vi "PSK 2 bit par symbole.vi"() -> ()   [LabVIEW 2010]
panel:
  out "signal demodulé":bool[](array[boolean])
  out "Signal Modulé":dynamicdata(graph)
  in  "Tableau":bool[](array[boolean])
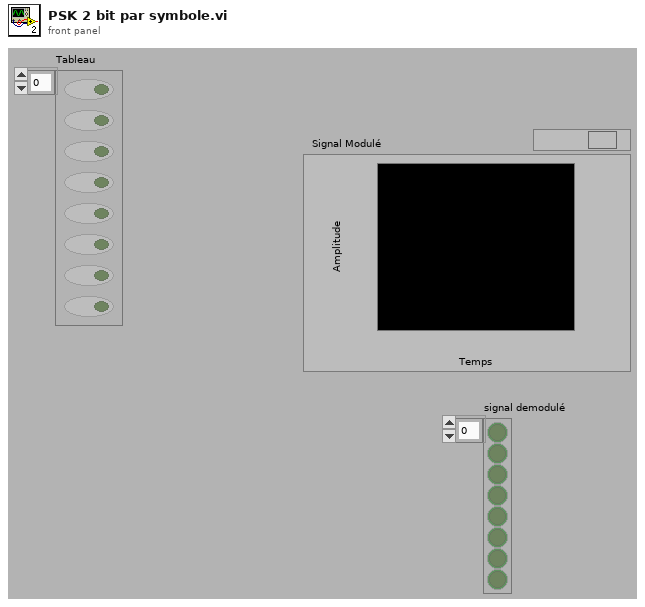
[diagram p1: front panel]
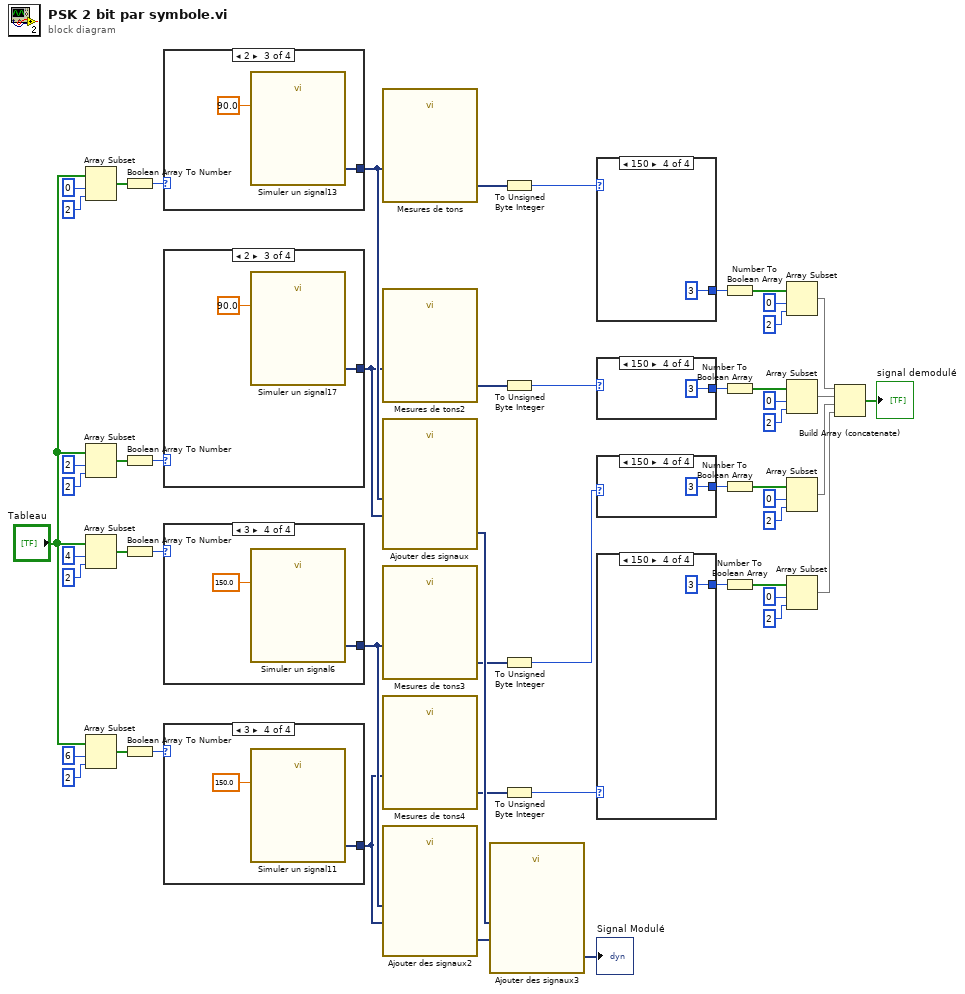
[diagram p0: block diagram]
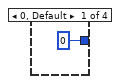
[diagram p2: hidden frame]
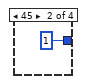
[diagram p3: hidden frame]
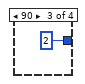
[diagram p4: hidden frame]
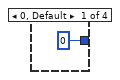
[diagram p5: hidden frame]
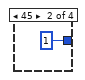
[diagram p6: hidden frame]
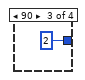
[diagram p7: hidden frame]
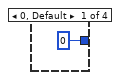
[diagram p8: hidden frame]
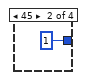
[diagram p9: hidden frame]
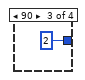
[diagram p10: hidden frame]
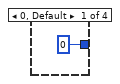
[diagram p11: hidden frame]
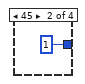
[diagram p12: hidden frame]
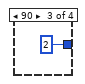
[diagram p13: hidden frame]
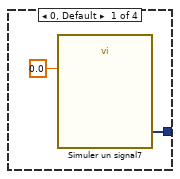
[diagram p14: hidden frame]
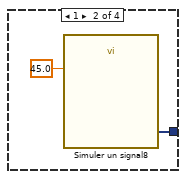
[diagram p15: hidden frame]
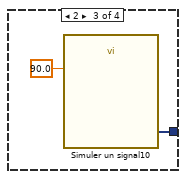
[diagram p16: hidden frame]
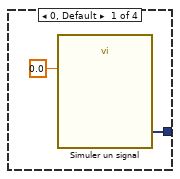
[diagram p17: hidden frame]
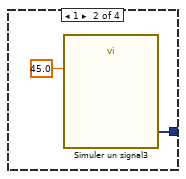
[diagram p18: hidden frame]
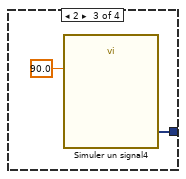
[diagram p19: hidden frame]
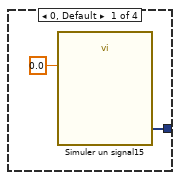
[diagram p20: hidden frame]
diagram:
  n1 = Array Subset(array="Tableau", index=0 ("indice"), length=2 ("longueur")) -> (w44:bool[])
  n2 = Array Subset(array="Tableau", index=2 ("indice"), length=2 ("longueur")) -> (w43:bool[])
  n3 = Array Subset(array="Tableau", index=4 ("indice"), length=2 ("longueur")) -> (w42:bool[])
  n4 = Array Subset(array="Tableau", index=6 ("indice"), length=2 ("longueur")) -> (w41:bool[])
  n5 = Boolean Array To Number(Boolean array=w44) -> (number=w40:u32)
  n6 = Boolean Array To Number(Boolean array=w43) -> (number=w38:u32)
  n7 = Boolean Array To Number(Boolean array=w42) -> (number=w36:u32)
  n8 = Boolean Array To Number(Boolean array=w41) -> (number=w35:u32)
  n9 = case shown="2" w40 {
    tunnel: [w54 w56 w58 w60] -> w33
    frame 0, Default {
      n10 = call "Simuler un signal5"("Phase"=0.0) -> ("Sinus"=w54:dynamicdata)  [unwired: 13 in, 1 out]
    }
    frame 1 {
      n11 = call "Simuler un signal9"("Phase"=45.0) -> ("Sinus"=w56:dynamicdata)  [unwired: 13 in, 1 out]
    }
    frame 2 {
      n12 = call "Simuler un signal13"("Phase"=90.0) -> ("Sinus"=w58:dynamicdata)  [unwired: 13 in, 1 out]
    }
    frame 3 {
      n13 = call "Simuler un signal2"("Phase"=150.0) -> ("Sinus"=w60:dynamicdata)  [unwired: 13 in, 1 out]
    }
  }
  n14 = case shown="2" w38 {
    tunnel: [w62 w64 w66 w68] -> w31
    frame 0, Default {
      n15 = call "Simuler un signal15"("Phase"=0.0) -> ("Sinus"=w62:dynamicdata)  [unwired: 13 in, 1 out]
    }
    frame 1 {
      n16 = call "Simuler un signal16"("Phase"=45.0) -> ("Sinus"=w64:dynamicdata)  [unwired: 13 in, 1 out]
    }
    frame 2 {
      n17 = call "Simuler un signal17"("Phase"=90.0) -> ("Sinus"=w66:dynamicdata)  [unwired: 13 in, 1 out]
    }
    frame 3 {
      n18 = call "Simuler un signal18"("Phase"=150.0) -> ("Sinus"=w68:dynamicdata)  [unwired: 13 in, 1 out]
    }
  }
  n19 = case shown="3" w36 {
    tunnel: [w70 w72 w74 w76] -> w30
    frame 0, Default {
      n20 = call "Simuler un signal"("Phase"=0.0) -> ("Sinus"=w70:dynamicdata)  [unwired: 13 in, 1 out]
    }
    frame 1 {
      n21 = call "Simuler un signal3"("Phase"=45.0) -> ("Sinus"=w72:dynamicdata)  [unwired: 13 in, 1 out]
    }
    frame 2 {
      n22 = call "Simuler un signal4"("Phase"=90.0) -> ("Sinus"=w74:dynamicdata)  [unwired: 13 in, 1 out]
    }
    frame 3 {
      n23 = call "Simuler un signal6"("Phase"=150.0) -> ("Sinus"=w76:dynamicdata)  [unwired: 13 in, 1 out]
    }
  }
  n24 = case shown="3" w35 {
    tunnel: [w78 w80 w82 w84] -> w29
    frame 0, Default {
      n25 = call "Simuler un signal7"("Phase"=0.0) -> ("Sinus"=w78:dynamicdata)  [unwired: 13 in, 1 out]
    }
    frame 1 {
      n26 = call "Simuler un signal8"("Phase"=45.0) -> ("Sinus"=w80:dynamicdata)  [unwired: 13 in, 1 out]
    }
    frame 2 {
      n27 = call "Simuler un signal10"("Phase"=90.0) -> ("Sinus"=w82:dynamicdata)  [unwired: 13 in, 1 out]
    }
    frame 3 {
      n28 = call "Simuler un signal11"("Phase"=150.0) -> ("Sinus"=w84:dynamicdata)  [unwired: 13 in, 1 out]
    }
  }
  n29 = call "Mesures de tons"("Signals"=w33) -> ("Phase"=w32:dynamicdata)  [unwired: 9 in, 1 out]
  n30 = call "Mesures de tons2"("Signals"=w31) -> ("Phase"=w27:dynamicdata)  [unwired: 9 in, 1 out]
  n31 = call "Ajouter des signaux"("Input Signal B"=w31, "Input Signal A"=w33) -> ("Appended Signals"=w39:dynamicdata)  [unwired: 8 in, 1 out]
  n32 = call "Mesures de tons3"("Signals"=w30) -> ("Phase"=w26:dynamicdata)  [unwired: 9 in, 1 out]
  n33 = call "Mesures de tons4"("Signals"=w29) -> ("Phase"=w28:dynamicdata)  [unwired: 9 in, 1 out]
  n34 = call "Ajouter des signaux2"("Input Signal B"=w29, "Input Signal A"=w30) -> ("Appended Signals"=w37:dynamicdata)  [unwired: 8 in, 1 out]
  n35 = call "Ajouter des signaux3"("Input Signal B"=w37, "Input Signal A"=w39) -> ("Appended Signals"=→"Signal Modulé":dynamicdata)  [unwired: 8 in, 1 out]
  n36 = To Unsigned Byte Integer(number=w32) -> (unsigned 8bit integer=w25:u8)
  n37 = To Unsigned Byte Integer(number=w27) -> (unsigned 8bit integer=w24:u8)
  n38 = To Unsigned Byte Integer(number=w26) -> (unsigned 8bit integer=w23:u8)
  n39 = To Unsigned Byte Integer(number=w28) -> (unsigned 8bit integer=w22:u8)
  n40 = case shown="150" w25 {
    tunnel: [0 1 2 3] -> w1
    frame 0, Default {
    }
    frame 45 {
    }
    frame 90 {
    }
    frame 150 {
    }
  }
  n41 = case shown="150" w24 {
    tunnel: [0 1 2 3] -> w19
    frame 0, Default {
    }
    frame 45 {
    }
    frame 90 {
    }
    frame 150 {
    }
  }
  n42 = case shown="150" w23 {
    tunnel: [0 1 2 3] -> w20
    frame 0, Default {
    }
    frame 45 {
    }
    frame 90 {
    }
    frame 150 {
    }
  }
  n43 = case shown="150" w22 {
    tunnel: [0 1 2 3] -> w21
    frame 0, Default {
    }
    frame 45 {
    }
    frame 90 {
    }
    frame 150 {
    }
  }
  n44 = Number To Boolean Array(number=w1) -> (Boolean array=w8:bool[])
  n45 = Number To Boolean Array(number=w19) -> (Boolean array=w11:bool[])
  n46 = Number To Boolean Array(number=w20) -> (Boolean array=w7:bool[])
  n47 = Number To Boolean Array(number=w21) -> (Boolean array=w16:bool[])
  n48 = Array Subset(array=w8, index=0 ("indice"), length=2 ("longueur")) -> (w6:bool[])
  n49 = Array Subset(array=w11, index=0 ("indice"), length=2 ("longueur")) -> (w5:bool[])
  n50 = Array Subset(array=w7, index=0 ("indice"), length=2 ("longueur")) -> (w4:bool[])
  n51 = Array Subset(array=w16, index=0 ("indice"), length=2 ("longueur")) -> (w3:bool[])
  n52 = Build Array (concatenate)(w6, w5, w4, w3) -> (→"signal demodulé":bool[])
